vi "Actor Core.vi"(8 "error in":errorcluster, 11 "Coffee Shop in":refnum<class "Coffee Shop.lvclass">) -> (0 "error out":errorcluster, 3 "Actor out":refnum<class "Actor.lvclass">)   [LabVIEW 2023, in "Coffee Shop.lvlib" / "Coffee Shop.lvclass"]
doc: "(<B>Filename</B>: Actor Framework.lvlib:Actor.lvclass:Actor Core.vi)\n\nReceives messages to the actor, reacts to them, and initiates any error handling that may shut the actor down.\n\nDescendant classes may override this VI to append parallel tasks for the actor to complete while it handles messages. Overrides use the Call Parent Method node."
uses:
  Coffee Shop.lvclass
  c:/dev/_r/4/eng/lv-core/lvpostprocessingd/lv_mc_x86_64/dist_i386/vi.lib/ActorFramework/Actor/Actor.lvclass
  <vilib>/ActorFramework/Actor/Actor.lvclass
  Status Display.ctl
  <vilib>/ActorFramework/Actor/Actor.lvclass/Actor.ctl
  <vilib>/ActorFramework/Message Enqueuer/Message Enqueuer.lvclass/Message Enqueuer.ctl
  Coffee Shop.lvclass/Coffee Shop.ctl
  Coffee Shop Messages/Remove Barista Msg/Remove Barista Msg.lvclass/Remove Barista Msg.ctl
  Coffee Shop Messages/Remove Customer Msg/Remove Customer Msg.lvclass/Remove Customer Msg.ctl
  Coffee Shop Messages/Remove Cashier Msg/Remove Cashier Msg.lvclass/Remove Cashier Msg.ctl
  Person Messages/Show or Hide Front Panel Msg/Show or Hide Front Panel Msg.lvclass
  c:/dev/_r/4/eng/lv-core/lvpostprocessingd/lv_mc_x86_64/dist_i386/vi.lib/ActorFramework/Message/Message.lvclass
  Entity Types.ctl
  Coffee Shop Messages/Fwd Message to Nested Actor Msg/Fwd Message to Nested Actor Msg.lvclass/Fwd Message to Nested Actor Msg.ctl
  <vilib>/ActorFramework/Message Enqueuer/Init from Existing Queue.vi
  <vilib>/ActorFramework/Message Enqueuer/Enqueue.vi
  <vilib>/ActorFramework/Stop Msg/Stop Msg.lvclass
  Coffee Shop Messages/Add Customer Msg/Add Customer Msg.lvclass
  Coffee Shop Messages/Add Cashier Msg/Add Cashier Msg.lvclass
  Coffee Shop Messages/Add Barista Msg/Add Barista Msg.lvclass
  Coffee Shop Messages/Remove Barista Msg/Remove Barista Msg.lvclass
  Coffee Shop Messages/Remove Customer Msg/Remove Customer Msg.lvclass
  Coffee Shop Messages/Remove Cashier Msg/Remove Cashier Msg.lvclass
  Coffee Shop Messages/Fwd Message to Nested Actor Msg/Fwd Message to Nested Actor Msg.lvclass
  <vilib>/ActorFramework/Message Priority Queue/Priority Enqueue.vi
  <vilib>/ActorFramework/Message Enqueuer/Message Enqueuer.lvclass
panel:
  in  "Remove Customer":bool
  in  "Stop Button":bool
  in  "Remove Barista":bool
  in  "Show Barista Info":bool
  in  "Add Barista":bool
  in  "Baristas":T1
  in  "Remove Cashier":bool
  in  "Show Cashier Info":bool
  in  "Add Cashier":bool
  in  "Cashiers":T1
  in  "Show Customer Info":bool
  in  "Add Customer":bool
  in  "Customers":T1
  # "Click + to add a customer actor to the system.\nClick Place Order to choose items for the customer to order.\nCustomer will wait until all items ordered are ready, then exit."
  # "Cashiers process orders into individual drink jobs and forwards those jobs to baristas.\nClick + to add a cashier actor to the system.\nClick - to remove a cashier from the system."
  # "Baristas process drink jobs and notify customers of completed drinks.\nAdd more baristas to the system by clicking +.  Pending jobs will be assigned to the next available barista.\nClick - to remove a barista from the system."
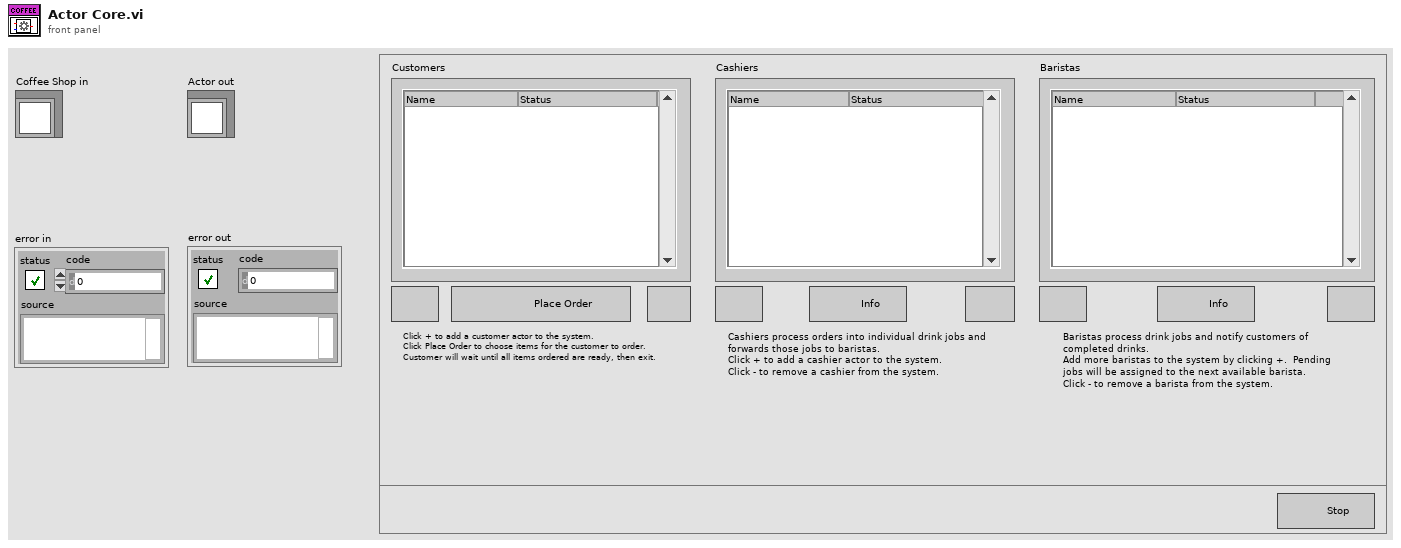
[diagram p1: front panel]
types:
  T1 = typedef "Coffee Shop.lvlib/Coffee Shop.lvclass/Status Display.ctl" = i32
  T2 = typedef "Coffee Shop.lvlib/Coffee Shop.lvclass/Entity Types.ctl" = enum16{"Customer", "Cashier", "Barista"}
  T3 = typedef "Entity Table.lvclass/Entity Types.ctl" = enum16{"Customer", "Cashier", "Barista"}
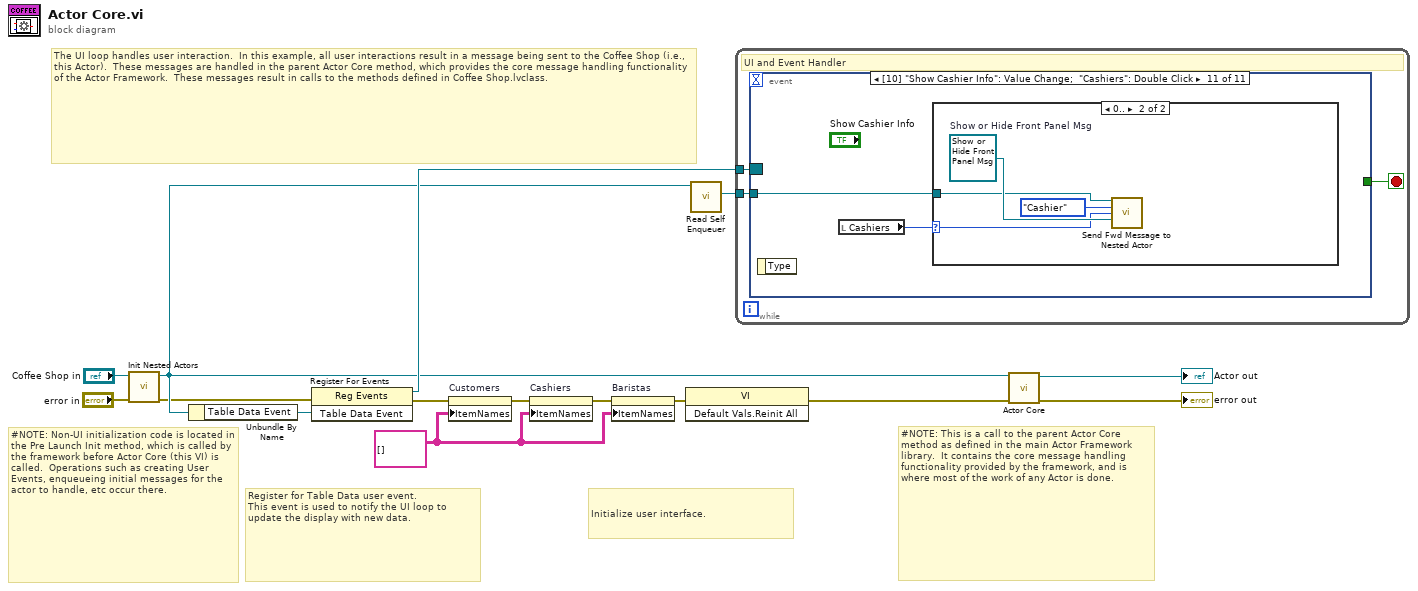
[diagram p0: block diagram]
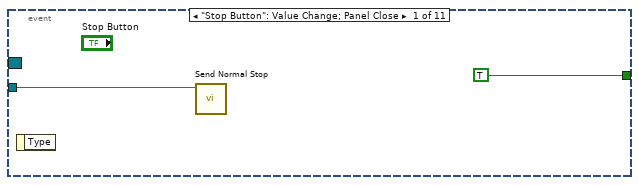
[diagram p2: hidden frame]
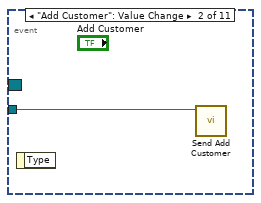
[diagram p3: hidden frame]
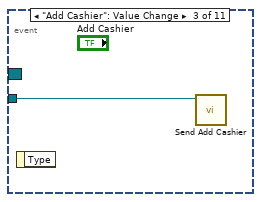
[diagram p4: hidden frame]
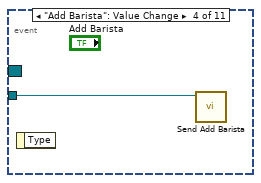
[diagram p5: hidden frame]
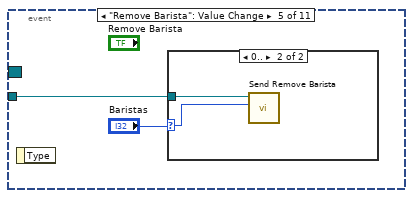
[diagram p6: hidden frame]
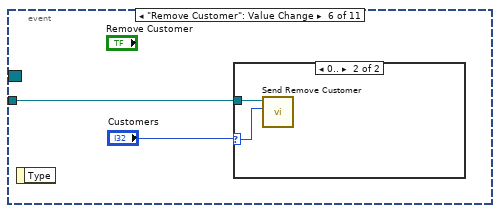
[diagram p8: hidden frame]
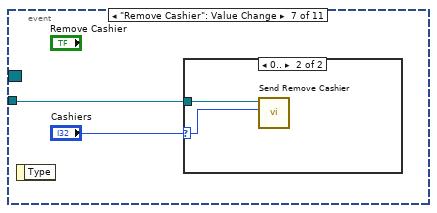
[diagram p10: hidden frame]
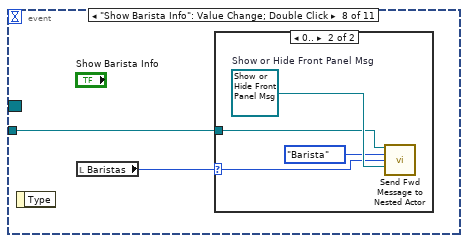
[diagram p12: hidden frame]
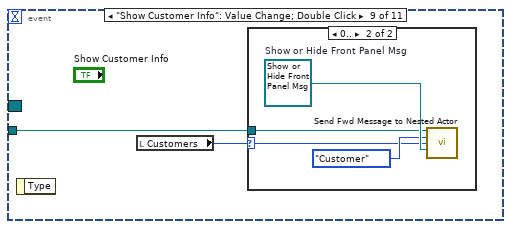
[diagram p14: hidden frame]
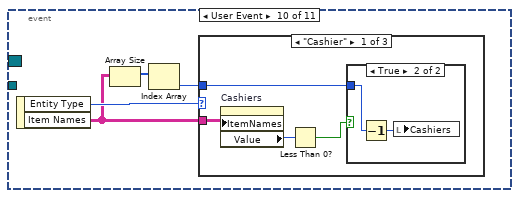
[diagram p16: hidden frame]
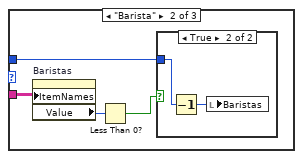
[diagram p18: hidden frame]
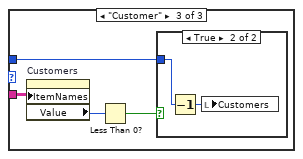
[diagram p20: hidden frame]
diagram:
  w13 = string[][] [] ("Item Names")
  # "#NOTE: Non-UI initialization code is located in the Pre Launch Init method, which is called by the framework before Actor Core (this VI) is called.  Operations such as creating User Events, enqueueing initial messages for the actor to handle, etc occur there."
  # "The UI loop handles user interaction.  In this example, all user interactions result in a message being sent to the Coffee Shop (i.e., this Actor).  These messages are handled in the parent Actor Core method, which provides the core message handling functionality of the Actor Framework.  These messages result in calls to the methods defined in Coffee Shop.lvclass."
  # "#NOTE: This is a call to the parent Actor Core method as defined in the main Actor Framework library.  It contains the core message handling functionality provided by the framework, and is where most of the work of any Actor is done."
  # "Register for Table Data user event.\nThis event is used to notify the UI loop to update the display with new data."
  # "Initialize user interface."
  n1 = call-dynamic "Init Nested Actors.vi"("error in (no error)"="error in", "Coffee Shop in"="Coffee Shop in") -> ("error out"=w1:errorcluster, "Coffee Shop out"=w3:refnum<class "Coffee Shop.lvclass">)  [unwired: 8 in]
  n2 = Unbundle By Name(w3) -> ("Table Data Event"=w6:refnum<user-event>)
  n3 = register-events(error in=w1, w6) -> (reference out=w5:refnum<event-registration>, error out=w8:errorcluster)  [unwired: 1 in]
  n4 = property on="Customers" class="MCListbox (strict)"(error in=w8, "ItemNames"=w13) -> (error out=w12:errorcluster)  [unwired: 1 in, 1 out]
  n5 = property on="Cashiers" class="MCListbox (strict)"(error in=w12, "ItemNames"=w13) -> (error out=w11:errorcluster)  [unwired: 1 in, 1 out]
  n6 = property on="Baristas" class="MCListbox (strict)"(error in=w11, "ItemNames"=w13) -> (error out=w7:errorcluster)  [unwired: 1 in, 1 out]
  n7 = invoke on="Invoke Node" class="VI" method="Default Vals.Reinit All"(error in=w7) -> (error out=w9:errorcluster)  [unwired: 2 in, 2 out]
  n8 = call <vilib>:"Read Self Enqueuer.vi"("Actor"=w3) -> ("Self Enqueuer"=w10:refnum<class "Message Enqueuer.lvclass">)  [unwired: 10 in]
  n9 = while {
    tunnel: w10 -> [w17]
    tunnel: w5 -> [w16]
    stop <- w18 stop-if-true
    # "UI and Event Handler"
    n10 = event shown="[10] \"Show Cashier Info\": Value Change;  \"Cashiers\": Double Click" {
      selector: w16 -> [_ _ _ _ _ _ _ _ _ _ _]
      dyn-events: _ -> [_ _ _ _ _ _ _ _ _ _ _]
      timeout: _ -> [_ _ _ _ _ _ _ _ _ _ _]
      tunnel: [TRUE ("Stop Button") _ _ _ _ _ _ _ _ _ _] -> w18
      tunnel: w17 -> [w19 w21 w22 w23 w25 w29 w33 w37 w43 _ w71]
      event "Stop Button": Value Change; Panel Close {
        n11 = event-data() -> ()  [unwired: 1 in, 1 out]
        n12 = call <vilib>:"Send Normal Stop.vi"("Message Enqueuer"=w19) -> ()  [unwired: 10 in, 1 out]
      }
      event "Add Customer": Value Change {
        n13 = event-data() -> ()  [unwired: 1 in, 1 out]
        n14 = call "Send Add Customer.vi"("Message Enqueuer"=w21) -> ()  [unwired: 9 in, 2 out]
      }
      event "Add Cashier": Value Change {
        n15 = event-data() -> ()  [unwired: 1 in, 1 out]
        n16 = call "Send Add Cashier.vi"("Message Enqueuer"=w22) -> ()  [unwired: 9 in, 2 out]
      }
      event "Add Barista": Value Change {
        n17 = event-data() -> ()  [unwired: 1 in, 1 out]
        n18 = call "Send Add Barista.vi"("Message Enqueuer"=w23) -> ()  [unwired: 9 in, 2 out]
      }
      event "Remove Barista": Value Change {
        n19 = event-data() -> ()  [unwired: 1 in, 1 out]
        n20 = case shown="0.." "Baristas" {
          selector: "Baristas" -> [_ w26]
          tunnel: w25 -> [_ w27]
          frame Default {
            # "Do not remove if no barista was selected"
          }
          frame 0.. {
            n21 = call "Send Remove Barista.vi"("Barista Index"=w26, "Message Enqueuer"=w27) -> ()  [unwired: 8 in, 2 out]
          }
        }
      }
      event "Remove Customer": Value Change {
        n22 = event-data() -> ()  [unwired: 1 in, 1 out]
        n23 = case shown="0.." "Customers" {
          selector: "Customers" -> [_ w30]
          tunnel: w29 -> [_ w31]
          frame Default {
            # "Do not remove if no customer was selected"
          }
          frame 0.. {
            n24 = call "Send Remove Customer.vi"("Customer Index"=w30, "Message Enqueuer"=w31) -> ()  [unwired: 8 in, 2 out]
          }
        }
      }
      event "Remove Cashier": Value Change {
        n25 = event-data() -> ()  [unwired: 1 in, 1 out]
        n26 = case shown="0.." "Cashiers" {
          selector: "Cashiers" -> [_ w34]
          tunnel: w33 -> [_ w35]
          frame Default {
            # "Do not remove if  no cashier was selected"
          }
          frame 0.. {
            n27 = call "Send Remove Cashier.vi"("Cashier Index"=w34, "Message Enqueuer"=w35) -> ()  [unwired: 8 in, 2 out]
          }
        }
      }
      event "Show Barista Info": Value Change; Double Click {
        n28 = event-data() -> ()  [unwired: 1 in, 1 out]
        n29 = local read "Baristas"() -> (w36:T1)
        n30 = case shown="0.." w36 {
          selector: w36 -> [_ w38]
          tunnel: w37 -> [_ w39]
          frame Default {
            # "Do nothing if no barista was selected"
          }
          frame 0.. {
            w41 = refnum<class "Show or Hide Front Panel Msg.lvclass"> refnum  # Show or Hide Front Panel Msg
            n31 = call "Send Fwd Message to Nested Actor.vi"("Message Enqueuer"=w39, "Entity Type"=Entity_Types."Barista", "Entity Index"=w38, "Message"=w41) -> ()  [unwired: 10 in, 2 out]
          }
        }
      }
      event "Show Customer Info": Value Change; Double Click {
        n32 = event-data() -> ()  [unwired: 1 in, 1 out]
        n33 = local read "Customers"() -> (w42:T1)
        n34 = case shown="0.." w42 {
          selector: w42 -> [_ w44]
          tunnel: w43 -> [_ w45]
          frame Default {
            # "Do nothing if no customer was selected"
          }
          frame 0.. {
            w47 = refnum<class "Show or Hide Front Panel Msg.lvclass"> refnum  # Show or Hide Front Panel Msg
            n35 = call "Send Fwd Message to Nested Actor.vi"("Message Enqueuer"=w45, "Entity Type"=Entity_Types."Customer", "Entity Index"=w44, "Message"=w47) -> ()  [unwired: 10 in, 2 out]
          }
        }
      }
      event User Event {
        n36 = event-data() -> ("Entity Type"=w51:T3, "Item Names"=w50:string[][])  [unwired: 1 in]
        n37 = Array Size(array=w50) -> (size(s)=w49:i32[])
        n38 = Index Array(array=w49) -> (element=w48:i32)  [unwired: 1 in]
        n39 = case shown="\"Cashier\"" w51 {
          tunnel: w50 -> [w55 w61 w67]
          tunnel: w48 -> [w53 w58 w64]
          frame "Cashier" {
            n40 = property on="Cashiers" class="MCListbox (strict)"("ItemNames"=w55) -> ("Value"=w52:T1)  [unwired: 2 in, 2 out]
            n41 = Less Than 0?(x=w52) -> (x < 0?=w54:bool)
            n42 = case shown="True" w54 {
              tunnel: w53 -> [_ w57]
              frame False {
              }
              frame True {
                n43 = Decrement(x=w57) -> (x-1=w56:i32)
                n44 = local write "Cashiers"(w56) -> ()
              }
            }
          }
          frame "Barista" {
            n45 = property on="Baristas" class="MCListbox (strict)"("ItemNames"=w61) -> ("Value"=w60:T1)  [unwired: 2 in, 2 out]
            n46 = Less Than 0?(x=w60) -> (x < 0?=w59:bool)
            n47 = case shown="True" w59 {
              tunnel: w58 -> [_ w63]
              frame False {
              }
              frame True {
                n48 = Decrement(x=w63) -> (x-1=w62:i32)
                n49 = local write "Baristas"(w62) -> ()
              }
            }
          }
          frame "Customer" {
            n50 = property on="Customers" class="MCListbox (strict)"("ItemNames"=w67) -> ("Value"=w66:T1)  [unwired: 2 in, 2 out]
            n51 = Less Than 0?(x=w66) -> (x < 0?=w65:bool)
            n52 = case shown="True" w65 {
              tunnel: w64 -> [_ w69]
              frame False {
              }
              frame True {
                n53 = Decrement(x=w69) -> (x-1=w68:i32)
                n54 = local write "Customers"(w68) -> ()
              }
            }
          }
        }
      }
      event "Show Cashier Info": Value Change; Double Click {
        n55 = event-data() -> ()  [unwired: 1 in, 1 out]
        n56 = local read "Cashiers"() -> (w70:T1)
        n57 = case shown="0.." w70 {
          selector: w70 -> [_ w72]
          tunnel: w71 -> [_ w73]
          frame Default {
            # "Do nothing if no cashier was selected"
          }
          frame 0.. {
            w75 = refnum<class "Show or Hide Front Panel Msg.lvclass"> refnum  # Show or Hide Front Panel Msg
            n58 = call "Send Fwd Message to Nested Actor.vi"("Message Enqueuer"=w73, "Entity Type"=Entity_Types."Cashier", "Entity Index"=w72, "Message"=w75) -> ()  [unwired: 10 in, 2 out]
          }
        }
      }
    }
  }
  n59 = call-parent "Actor Core.vi"("error in"=w9, "Actor in"=w3) -> ("error out"=→"error out":errorcluster, "Actor out"=→"Actor out":refnum<class "Actor.lvclass">)  [unwired: 8 in]
